vi "Show status message.vi"(8 "error in (no error)":errorcluster, 11 "Status Message":string) -> (0 "error out":errorcluster)   [LabVIEW 2013]
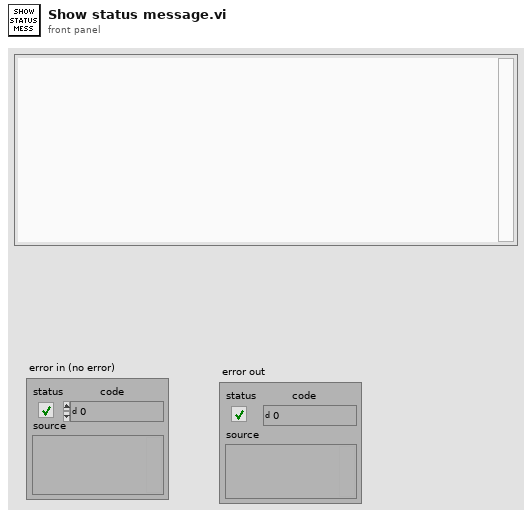
[diagram p1: front panel]
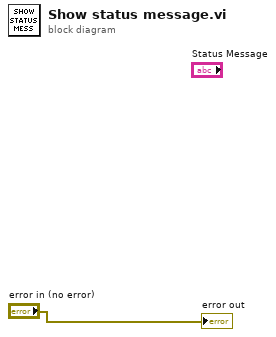
[diagram p0: block diagram]
diagram:
  "error out" <- "error in (no error)"
